vi "drot - Givens Rotation (DBL).vi"(5 "yInc":i32=1, 7 "xInc":i32=1, 8 "s":dbl, 9 "c":dbl=1.0, 10 "y in":dbl[](array[numeric]), 11 "x in":dbl[](array[numeric])) -> (0 "error":i32, 2 "y out":dbl[](array[numeric]), 3 "x out":dbl[](array[numeric]))   [LabVIEW 2020, in "NI_AALBLAS.lvlib"]
doc: "Applies a Givens rotation to a set of points."
uses:
  NI_AALBLAS.lvlib
  Fucntion.ctl
  BLAS1 Utility(DBL).vi
panel:
  # "x out(i)=c*x in(i)+s*y in(i)\ny out(i)=c*y in(i)-s*x in(i)"
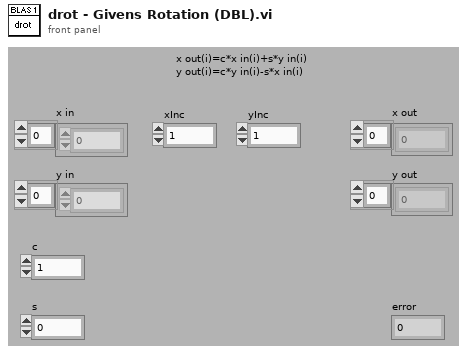
[diagram p1: front panel]
types:
  T1 = typedef "NI_AALBLAS.lvlib/Fucntion.ctl" = u16
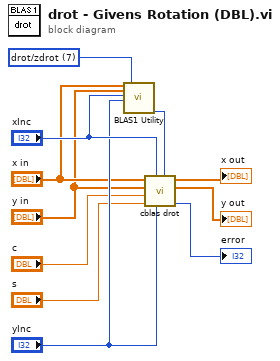
[diagram p0: block diagram]
diagram:
  w3 = T1 7 items=["ddot/zdotu/zdotc", "daxpy/zaxpy", "dnrm2/dznrm2", "dasum/dzasum", "dcopy/zcopy", "dswap/zswap", "drotm", "drot/zdrot", "idamax/izamax", "idamin/izamin", "dgemv/zgemv", "dsymv/zhemv", "dtrmv/ztrmv", "dsyr/zher", "dsyr2/zher2", "dger/zgeru/zgerc", "dtrsv/ztrsv", "dgemm/zgemm", "dsymm/zsymm/zhemm", "dtrmm/ztrmm", "dsyrk/zsyrk/zherk", "dsyr2k/zsyr2k/zher2k", "dtrsm/ztrsm"] ("function")
  n1 = call-poly "BLAS1 Utility.vi"("x"="x in", "y"="y in", "xInc"="xInc", "yInc"="yInc", "function"=w3) -> ("n"=w2:i32)  [unwired: 14 out]
  n2 = call "cblas drot.vi"("n"=w2, "incy"="yInc", "incx"="xInc", "s"="s", "c"="c", "y in"="y in", "x in"="x in") -> ("error"=→"error":i32, "y out"=→"y out":dbl[], "x out"=→"x out":dbl[])  [unwired: 2 out]
